vi "Main.vi"(8 "error in":errorcluster, 11 "AnotherWorkers in":refnum<class "AnotherWorkers.lvclass">) -> (0 "error out":errorcluster, 3 "AnotherWorkers out":refnum<class "AnotherWorkers.lvclass">)   [LabVIEW 2025, in "AnotherWorkers.lvclass"]
doc: "The <b>Queued Message Handler</b> of the Worker that owns this VI."
uses:
  AnotherWorkers.lvclass
  C:/Program Files (x86)/National Instruments/LabVIEW 2025/vi.lib/addons/_Workers/Library/Classes/Worker/Worker.lvclass
  Initialization Data.ctl
  Response Cases.ctl
  <vilib>/addons/_Workers/Library/Case Label.ctl
  AnotherWorkers.lvclass/AnotherWorkers.ctl
  rqp_GenerateRandomNumber.ctl
  rwr_ReturnRandomNumber.ctl
  rwr_ReturnRandomNumber Reply.ctl
  rqp_GeneratePasswordKey.ctl
  rsp_ReturnPasswordKey.ctl
  <vilib>/numeric/Random Number (Range) DBL.vi
  89fe8186-e2c8-4eb4-a2f1-b944d8fc450f.vi
  <vilib>/numeric/Random Number (Range) U64.vi
  <vilib>/numeric/sub_Random U32.vi
  <vilib>/addons/_Workers/Library/Classes/Message Queue/Message Queue.lvclass
  <vilib>/addons/_Workers/Library/Workers.lvlib
  993992fb-1281-40bc-abca-54ab46beb288.vi
panel:
  out "RandomNum_Response":u64
  out "RandomNum_wtihReply":dbl
  out "RandomNum":dbl
  # "Another Workers"
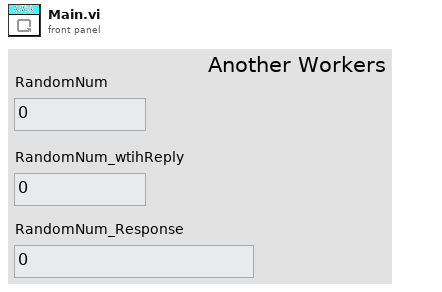
[diagram p1: front panel]
types:
  T1 = typedef "AnotherWorkers.lvclass/Initialization Data.ctl" = cluster{"Response Cases":T2}
  T2 = typedef "AnotherWorkers.lvclass/Response Cases.ctl" = cluster{"Placeholder - Can be deleted":string, "ReturnPasswordKey":T3}
  T3 = typedef "Workers.lvlib/Case Label.ctl" = string
  T4 = typedef "AnotherWorkers.lvclass/rqp_GenerateRandomNumber.ctl" = cluster{"String":string}
  T5 = typedef "AnotherWorkers.lvclass/rwr_ReturnRandomNumber Reply.ctl" = cluster{"String":string}
  T6 = typedef "AnotherWorkers.lvclass/rwr_ReturnRandomNumber.ctl" = cluster{"String":string}
  T7 = typedef "AnotherWorkers.lvclass/rsp_ReturnPasswordKey.ctl" = cluster{"String":string}
  T8 = typedef "AnotherWorkers.lvclass/rqp_GeneratePasswordKey.ctl" = cluster{"String":string}
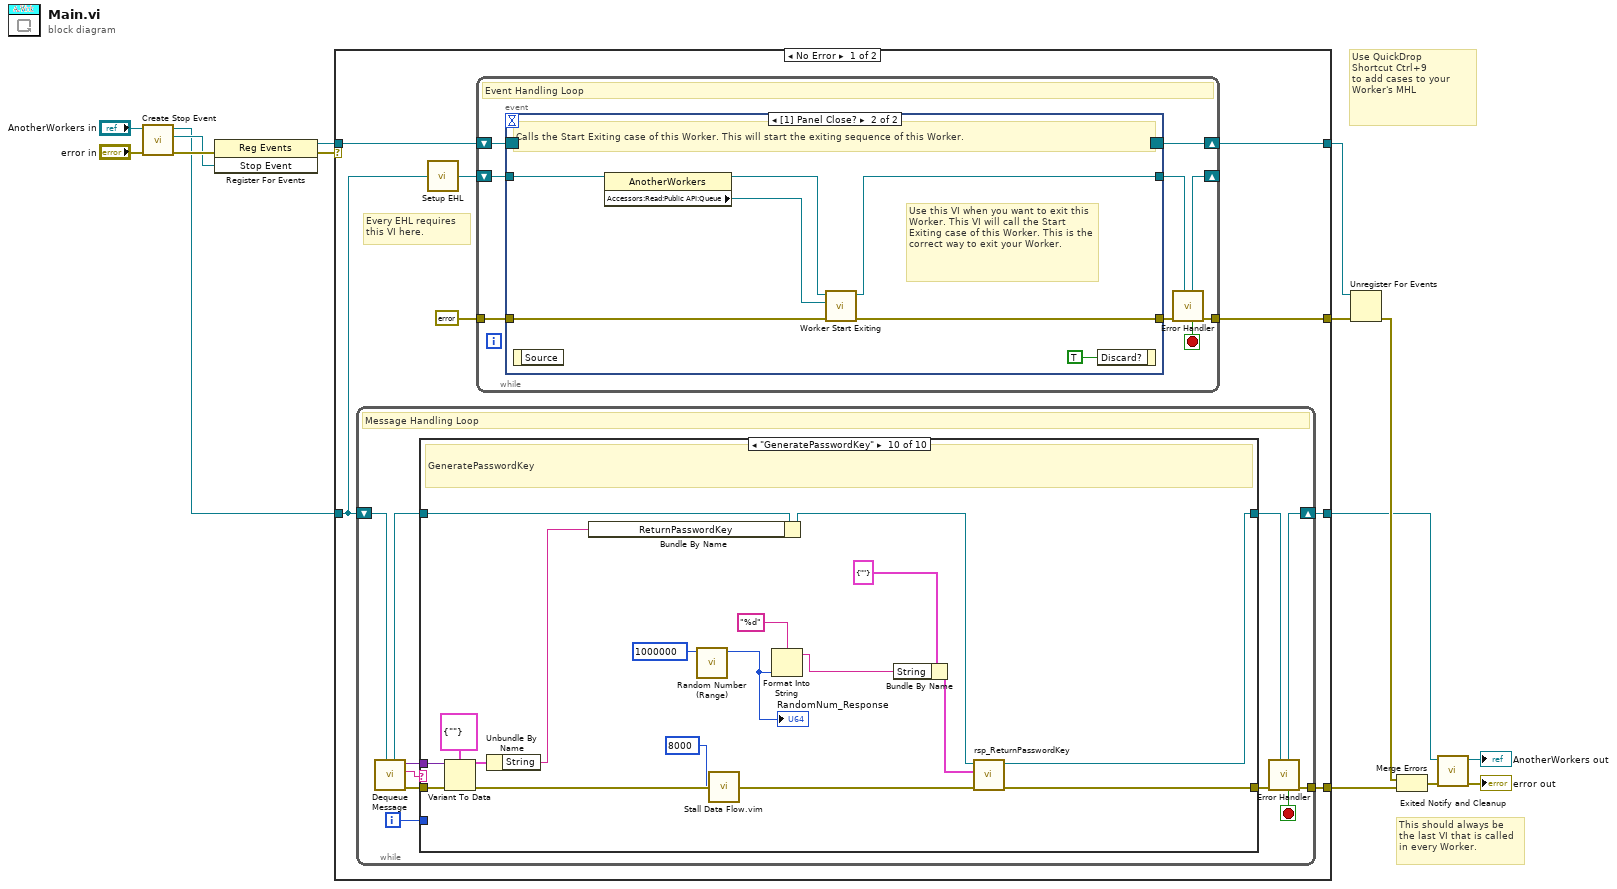
[diagram p0: block diagram]
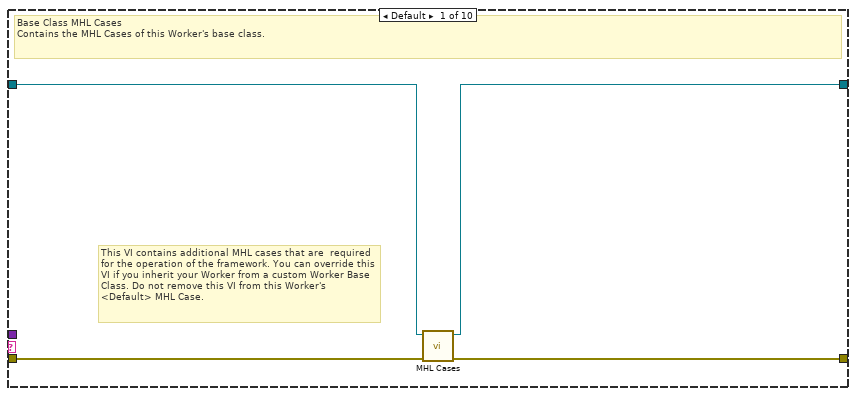
[diagram p2: hidden frame]
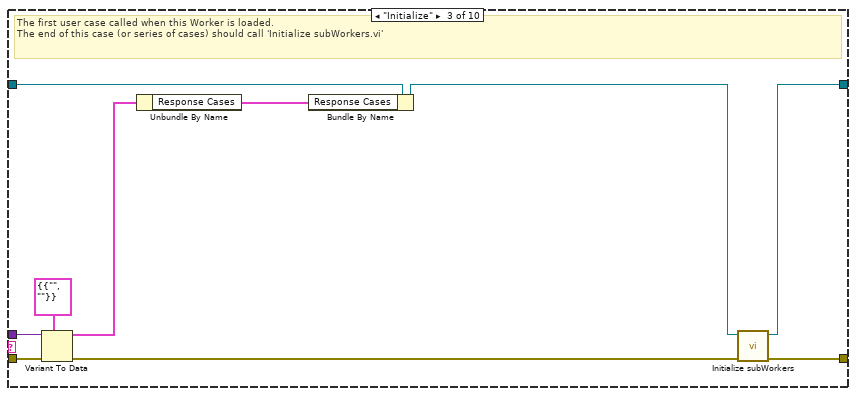
[diagram p4: hidden frame]
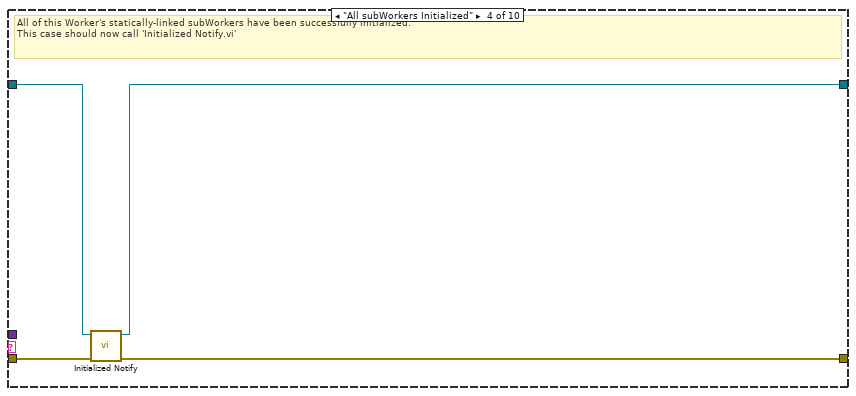
[diagram p5: hidden frame]
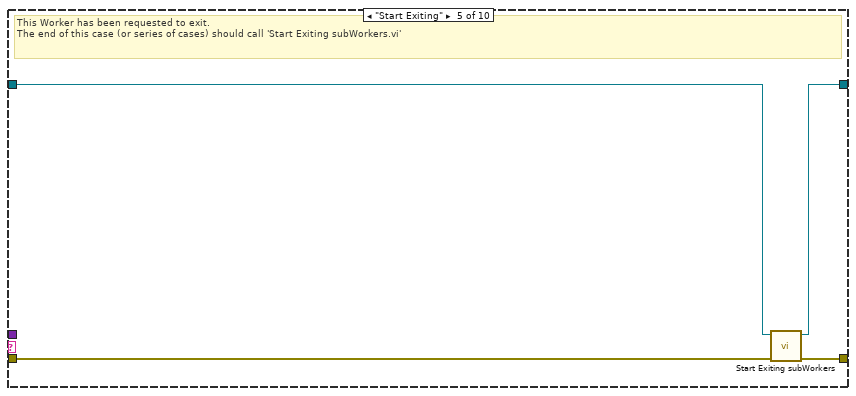
[diagram p6: hidden frame]
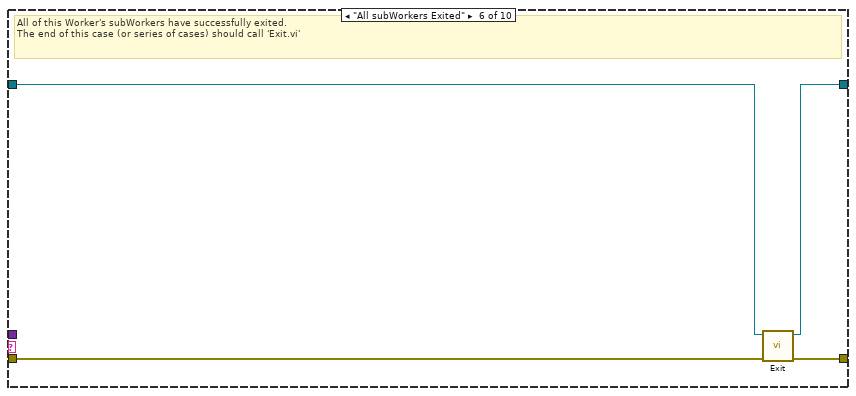
[diagram p7: hidden frame]
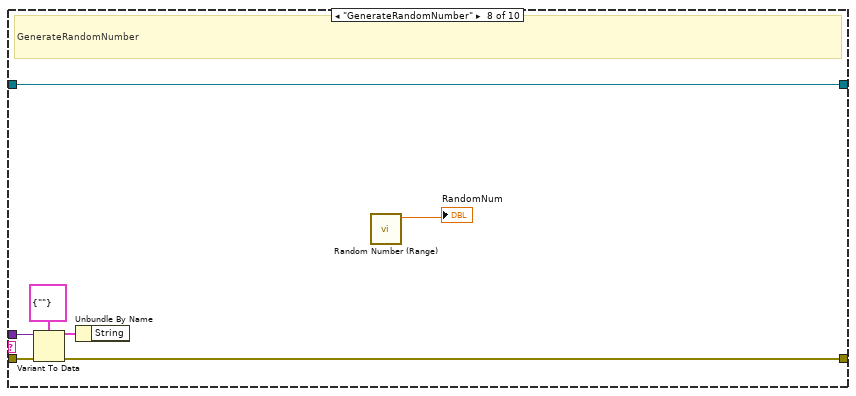
[diagram p9: hidden frame]
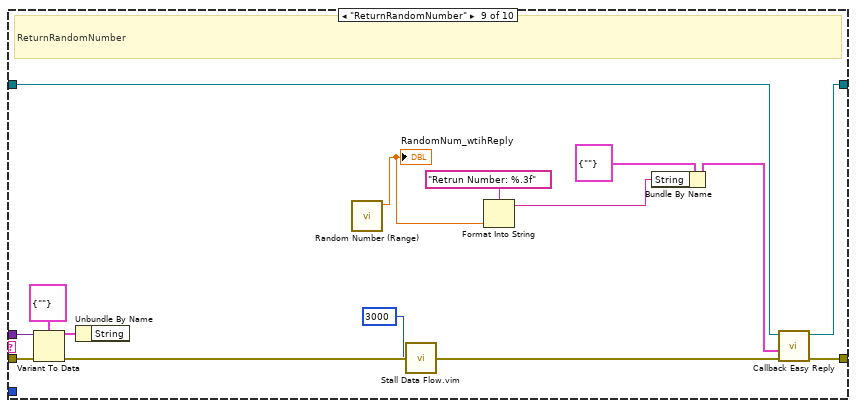
[diagram p10: hidden frame]
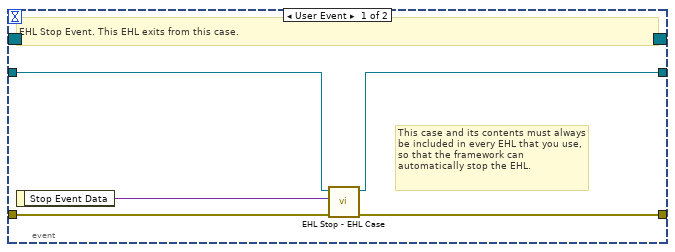
[diagram p11: hidden frame]
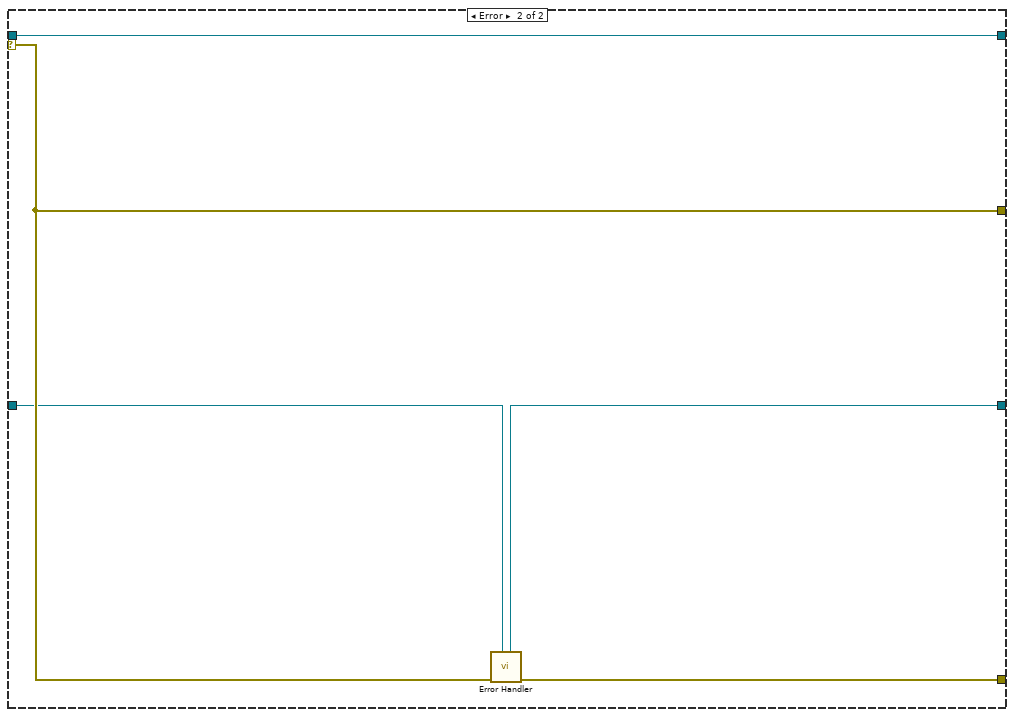
[diagram p12: hidden frame]
diagram:
  # "Use QuickDrop\nShortcut Ctrl+9\nto add cases to your\nWorker's MHL"
  # "This should always be the last VI that is called in every Worker."
  n1 = call-dynamic "Create Stop Event.vi"("error in"="error in", "Worker"="AnotherWorkers in") -> ("error out"=w10:errorcluster, "Stop Event"=w7:refnum<user-event>, "Worker out"=w4:refnum<class "AnotherWorkers.lvclass">)  [unwired: 7 in]
  n2 = register-events(error in=w10, w7) -> (reference out=w9:refnum<event-registration>, error out=w1:errorcluster)  [unwired: 1 in]
  n3 = case shown="No Error" w1 {
    tunnel: w4 -> [w18 w127]
    tunnel: [w16 w128] -> w8
    tunnel: w9 -> [w23 w129]
    tunnel: [w20 w130] -> w14
    tunnel: [w22 w129] -> w13
    tunnel: [w17 w126] -> w11
    selector: w1 -> [_ w130]
    frame No Error {
      # "Every EHL requires\nthis VI here."
      n4 = while {
        shift-right: [w32] -> w17
        shift-left: w18 -> [w34]
        tunnel: [w33] -> w16
        i -> [w25]
        stop <- w26 stop-if-true
        # "Message Handling Loop"
        n5 = call-dynamic "Dequeue Message.vi"("Worker"=w34) -> ("error out"=w31:errorcluster, "Case out"=w27:string, "Data out"=w24:variant, "Worker out"=w29:refnum<class "AnotherWorkers.lvclass">)  [unwired: 6 in, 1 out]
        n6 = case "Worker MHL Case Structure (DO NOT CHANGE LABEL NAME)" shown="\"GeneratePasswordKey\"" w27 {
          tunnel: w31 -> [w38 w39 w48 w52 w55 w62 w64 w70 w86 w104]
          tunnel: [w37 w39 w50 w51 w58 w61 w64 w69 w81 w97] -> w30
          tunnel: w29 -> [w36 w40 w47 w54 w56 w60 w63 w71 w79 w96]
          tunnel: [w35 w40 w49 w53 w57 w59 w63 w71 w80 w95] -> w28
          tunnel: w25 -> [_ _ _ _ _ _ _ _ _ _]
          tunnel: w24 -> [_ _ w45 _ _ _ _ w67 w83 w101]
          frame Default {
            # "This VI contains additional MHL cases that are  required for the operation of the framework. You can override this VI if you inherit your Worker from a custom Worker Base Class. Do not remove this VI from this Worker's <Default> MHL Case."
            # "Base Class MHL Cases\nContains the MHL Cases of this Worker's base class."
            n7 = call-dynamic "MHL Cases.vi"("error in"=w38, "Worker in"=w36) -> ("error out"=w37:errorcluster, "Worker out"=w35:refnum<class "AnotherWorkers.lvclass">)  [unwired: 8 in]
          }
          frame "------------ FRAMEWORK CASES -----------" {
            # "Start of Workers Framework Cases"
          }
          frame "Initialize" {
            # "The first user case called when this Worker is loaded.\nThe end of this case (or series of cases) should call 'Initialize subWorkers.vi'"
            n8 = Variant To Data(error in=w48, type=T1 {"Response Cases"={"Placeholder - Can be deleted"="", "ReturnPasswordKey"=""}} ("Initialization Data"), Variant=w45) -> (data=w43:T1, error out=w46:errorcluster)
            n9 = Unbundle By Name(w43) -> ("Response Cases"=w42:T2)
            n10 = Bundle By Name(cluster=w47, "Response Cases"=w42) -> (w44:refnum<class "AnotherWorkers.lvclass">)
            n11 = call-dynamic "Initialize subWorkers.vi"("error in"=w46, "Worker"=w44) -> ("error out"=w50:errorcluster, "dup Worker out"=w49:refnum<class "AnotherWorkers.lvclass">)  [unwired: 8 in]
          }
          frame "All subWorkers Initialized" {
            # "All of this Worker's statically-linked subWorkers have been successfully initialized.\nThis case should now call 'Initialized Notify.vi'"
            n12 = call-dynamic "Initialized Notify.vi"("error in"=w52, "Worker"=w54) -> ("error out"=w51:errorcluster, "dup Worker out"=w53:refnum<class "AnotherWorkers.lvclass">)  [unwired: 8 in]
          }
          frame "Start Exiting" {
            # "This Worker has been requested to exit. \nThe end of this case (or series of cases) should call 'Start Exiting subWorkers.vi'"
            n13 = call-dynamic "Start Exiting subWorkers.vi"("error_in"=w55, "Worker"=w56) -> ("error out"=w58:errorcluster, "dup Worker out"=w57:refnum<class "AnotherWorkers.lvclass">)  [unwired: 8 in]
          }
          frame "All subWorkers Exited" {
            # "All of this Worker's subWorkers have successfully exited. \nThe end of this case (or series of cases) should call 'Exit.vi'"
            n14 = call-dynamic "Exit.vi"("error_in"=w62, "Worker"=w60) -> ("error out"=w61:errorcluster, "dup Worker out"=w59:refnum<class "AnotherWorkers.lvclass">)  [unwired: 8 in]
          }
          frame "------------- PUBLIC API CASES -------------" {
            # "Start of Workers Public API Cases"
          }
          frame "GenerateRandomNumber" {
            # "GenerateRandomNumber"
            n15 = Variant To Data(error in=w70, type=T4 {"String"=""} ("Data"), Variant=w67) -> (data=w66:T4, error out=w69:errorcluster)
            n16 = Unbundle By Name(w66) -> ()  [unwired: 1 out]
            n17 = call-poly <vilib>:"Random Number (Range).vi"() -> ("number"=→"RandomNum":dbl)  [unwired: 11 in]
          }
          frame "ReturnRandomNumber" {
            # "ReturnRandomNumber"
            n18 = Variant To Data(error in=w86, type=T6 {"String"=""} ("Data"), Variant=w83) -> (data=w82:T6, error out=w85:errorcluster)
            n19 = Unbundle By Name(w82) -> ()  [unwired: 1 out]
            n20 = call-poly <vilib>:"Random Number (Range).vi"() -> ("number"=w76:dbl)  [unwired: 11 in]
            "RandomNum_wtihReply" <- w76
            n21 = call "Stall Data Flow.vim"("value in"=w85, "milliseconds to wait"=u32 3000) -> ("value out"=w73:errorcluster)  [unwired: 1 out]
            n22 = Format Into String(format string="Retrun Number: %.3f", w76) -> (resulting string=w74:string)  [unwired: 2 in, 1 out]
            n23 = Bundle By Name(cluster=T5 {"String"=""} ("Reply Data"), "String"=w74) -> (w77:T5)
            n24 = call-dynamic "Callback Easy Reply.vi"("error in"=w73, "Data"=w77, "Worker"=w79) -> ("error out"=w81:errorcluster, "dup Worker out"=w80:refnum<class "AnotherWorkers.lvclass">)  [unwired: 7 in]
          }
          frame "GeneratePasswordKey" {
            # "GeneratePasswordKey"
            n25 = Variant To Data(error in=w104, type=T8 {"String"=""} ("Data"), Variant=w101) -> (data=w100:T8, error out=w103:errorcluster)
            n26 = Unbundle By Name(w100) -> ("String"=w87:string)
            n27 = Bundle By Name(cluster=w96, "ReturnPasswordKey"=w87) -> (w88:refnum<class "AnotherWorkers.lvclass">)
            n28 = call-poly <vilib>:"Random Number (Range).vi"("upper bound (100)"=u64 1000000) -> ("number"=w91:u64)  [unwired: 10 in]
            "RandomNum_Response" <- w91
            n29 = call "Stall Data Flow.vim"("value in"=w103, "milliseconds to wait"=u32 8000) -> ("value out"=w90:errorcluster)  [unwired: 1 out]
            n30 = Format Into String(format string="%d", w91) -> (resulting string=w92:string)  [unwired: 2 in, 1 out]
            n31 = Bundle By Name(cluster=T7 {"String"=""} ("Data in"), "String"=w92) -> (w93:T7)
            n32 = call "rsp_ReturnPasswordKey.vi"("error in"=w90, "Data in"=w93, "AnotherWorkers in"=w88) -> ("error out"=w97:errorcluster, "dup AnotherWorkers out"=w95:refnum<class "AnotherWorkers.lvclass">)  [unwired: 7 in]
          }
        }
        n33 = call-dynamic "Error Handler.vi"("Worker"=w28, "error_in"=w30) -> ("error out"=w33:errorcluster, "Stop Loop"=w26:bool, "Worker out"=w32:refnum<class "AnotherWorkers.lvclass">)  [unwired: 7 in]
      }
      n34 = call-dynamic "Setup EHL.vi"("Worker"=w18) -> ("Worker out"=w19:refnum<class "AnotherWorkers.lvclass">)  [unwired: 14 in]
      n35 = while "Event Handling Loop" {
        shift-right: [w113] -> w22
        shift-left: w23 -> [w112]
        tunnel: [w108] -> w20
        tunnel: errorcluster {"status"=FALSE, "code"=0, "source"=""} ("error constant") -> [w110]
        shift-right: [w106] -> _
        shift-left: w19 -> [w111]
        stop <- w105 stop-if-true
        # "Event Handling Loop"
        n36 = event shown="[1] Panel Close?" {
          selector: w112 -> [_ _]
          dyn-events: [_ _] -> w113
          timeout: _ -> [_ _]
          tunnel: [w117 w124] -> w109
          tunnel: w110 -> [w118 w123]
          tunnel: w111 -> [w116 w122]
          tunnel: [w115 w121] -> w107
          event User Event {
            # "This case and its contents must always be included in every EHL that you use, so that the framework can automatically stop the EHL."
            # "EHL Stop Event. This EHL exits from this case."
            n37 = event-data() -> ("Stop Event Data"=w114:variant)  [unwired: 1 in]
            n38 = call-dynamic "EHL Stop - EHL Case.vi"("error in"=w118, "Stop Event Data"=w114, "Worker"=w116) -> ("error out"=w117:errorcluster, "Worker out"=w115:refnum<class "AnotherWorkers.lvclass">)  [unwired: 7 in]
          }
          event Panel Close? {
            # "Use this VI when you want to exit this Worker. This VI will call the Start Exiting case of this Worker. This is the correct way to exit your Worker."
            # "Calls the Start Exiting case of this Worker. This will start the exiting sequence of this Worker."
            n39 = event-data() -> ()  [unwired: 1 in, 1 out]
            n40 = property class="AnotherWorkers"(reference=w122) -> (reference out=w120:refnum<class "AnotherWorkers.lvclass">, "Accessors:Read:Public API:Queue"=w119:refnum<class "Message Queue.lvclass">)  [unwired: 1 in, 1 out]
            n41 = call-dynamic "Worker Start Exiting.vi"("error_in"=w123, "Message Queue"=w119, "Worker"=w120) -> ("error out"=w124:errorcluster, "dup Worker out"=w121:refnum<class "AnotherWorkers.lvclass">)  [unwired: 7 in]
            n42 = event-data("Discard?"=TRUE) -> ()  [unwired: 1 in, 1 out]
          }
        }
        n43 = call-dynamic "Error Handler.vi"("Worker"=w107, "error_in"=w109) -> ("error out"=w108:errorcluster, "Stop Loop"=w105:bool, "Worker out"=w106:refnum<class "AnotherWorkers.lvclass">)  [unwired: 7 in]
      }
    }
    frame Error {
      n44 = call-dynamic "Error Handler.vi"("Worker"=w127, "error_in"=w130) -> ("error out"=w128:errorcluster, "Worker out"=w126:refnum<class "AnotherWorkers.lvclass">)  [unwired: 7 in, 1 out]
    }
  }
  n45 = Unregister For Events(event registration refnum=w13, error in=w14) -> (error out=w15:errorcluster)
  n46 = Merge Errors(w15, w8) -> (w12:errorcluster)
  n47 = call-dynamic "Exited Notify and Cleanup.vi"("error_in"=w12, "Worker"=w11) -> ("error out"=→"error out":errorcluster, "dup Worker out"=→"AnotherWorkers out":refnum<class "AnotherWorkers.lvclass">)  [unwired: 8 in]
